vi "PH_Beamline.set start page.vi"(0 "i ref in":refnum<vi>, 2 "Tab Control Ref":refnum<vi>, 5 "error in (no error)":errorcluster) -> (14 "i ref out":refnum<vi>, 19 "error out":errorcluster)   [LabVIEW 2014, in "PH_Beamline.lvlib"]
uses:
  PH_Beamline.lvlib
  CSCore/CSSystem/CSSystemLib/CSSystemLib.lvlib
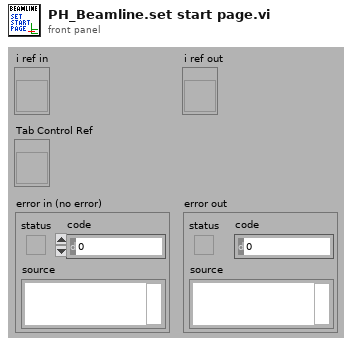
[diagram p1: front panel]
types:
  T1 = enum32{"ns-Frontend", "fs-Frontend", "PreAmp", "PA ED", "In.-Box", "MainAmp", "MAS", "Booster", "Comp", "Exp", "Mirrortower"}
  T2 = enum32{"ns-FE", "fs-FE", "uOPA", "PA", "PA ED", "In.-Box", "MainAmp", "MAS", "Booster", "Comp", "Exp", "Mirrortower", "Laserlab"}
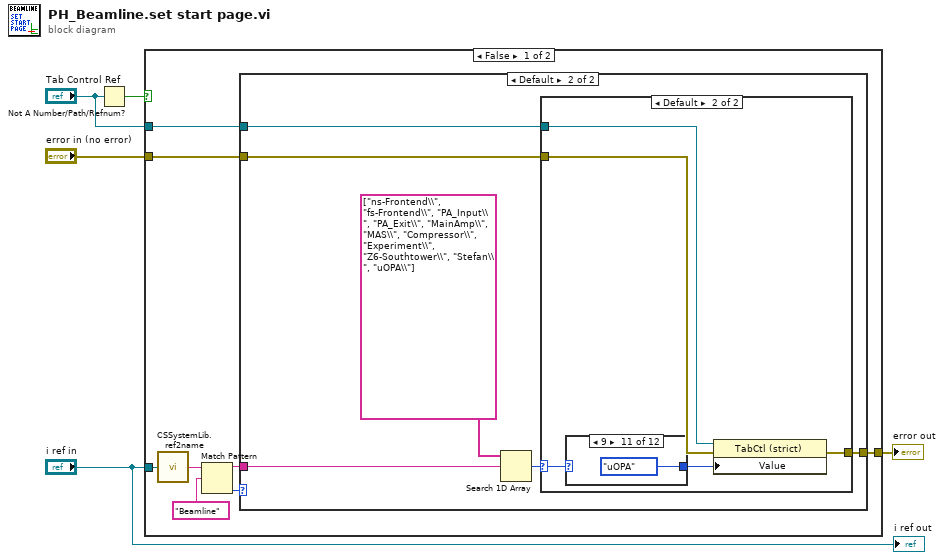
[diagram p0: block diagram]
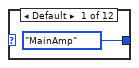
[diagram p4: hidden frame]
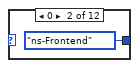
[diagram p5: hidden frame]
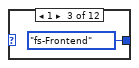
[diagram p6: hidden frame]
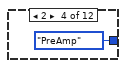
[diagram p7: hidden frame]
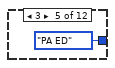
[diagram p8: hidden frame]
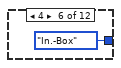
[diagram p9: hidden frame]
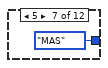
[diagram p10: hidden frame]
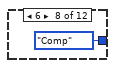
[diagram p11: hidden frame]
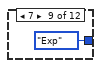
[diagram p12: hidden frame]
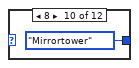
[diagram p13: hidden frame]
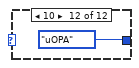
[diagram p14: hidden frame]
diagram:
  n1 = Not A Number/Path/Refnum?(number/path/refnum="Tab Control Ref") -> (NaN/Path/Refnum?=w2:bool)
  n2 = case shown="False" w2 {
    tunnel: "i ref in" -> [w13 _]
    tunnel: "Tab Control Ref" -> [w8 _]
    tunnel: [w7 w39] -> w4
    tunnel: "error in (no error)" -> [w6 w39]
    frame False {
      n3 = call "CSSystemLib.ref2name.vi"("obj refnum"=w13) -> ("name"=w9:string)
      n4 = Match Pattern(string=w9, regular expression="Beamline") -> (before substring=w11:string, offset past match=w12:i32)  [unwired: 1 in, 2 out]
      n5 = case shown="Default" w12 {
        tunnel: w11 -> [_ w15]
        tunnel: w8 -> [_ w18]
        tunnel: [w14 w17] -> w7
        tunnel: w6 -> [w14 w16]
        frame -1 {
        }
        frame Default {
          n6 = Search 1D Array(1D array=string[] ["ns-Frontend\\", "fs-Frontend\\", "PA_Input\\", "PA_Exit\\", "MainAmp\\", "MAS\\", "Compressor\\", "Experiment\\", "Z6-Southtower\\", "Stefan\\", "uOPA\\"], element=w15) -> (index of element=w19:i32)  [unwired: 1 in]
          n7 = case shown="Default" w19 {
            selector: w19 -> [_ w23]
            tunnel: w18 -> [_ w26]
            tunnel: [w21 w25] -> w17
            tunnel: w16 -> [w21 w24]
            frame -1 {
            }
            frame Default {
              n8 = case shown="9" w23 {
                tunnel: [T1."MainAmp" ("Tab Control") T1."ns-Frontend" ("Tab Control") T1."fs-Frontend" ("Tab Control") T1."PreAmp" ("Tab Control") T1."PA ED" ("Tab Control") T1."In.-Box" ("Tab Control") T1."MAS" ("Tab Control") T1."Comp" ("Tab Control") T1."Exp" ("Tab Control") T1."Mirrortower" ("Tab Control") T2."uOPA" ("Value") T2."uOPA" ("Value")] -> w22
                frame Default {
                }
                frame 0 {
                }
                frame 1 {
                }
                frame 2 {
                }
                frame 3 {
                }
                frame 4 {
                }
                frame 5 {
                }
                frame 6 {
                }
                frame 7 {
                }
                frame 8 {
                }
                frame 9 {
                }
                frame 10 {
                }
              }
              n9 = property on="Property Node" class="TabCtl (strict)"(reference=w26, error in=w24, "Value"=w22) -> (error out=w25:errorcluster)  [unwired: 1 out]
            }
          }
        }
      }
    }
    frame True {
    }
  }
  "error out" <- w4
  "i ref out" <- "i ref in"
